vi "averageMeasures.vi"(6 "shift_step_us":dbl=25.0 caption="Shift step", 8 "delay_us":dbl caption="Delay", 9 "repetitions":i32, 11 "counts":u32[][](array[numeric])) -> (2 "delays":dbl[](array[numeric]), 3 "counts":dbl[][](array[numeric]))   [LabVIEW 2014]
uses:
  <vilib>/Analysis/baseanly.llb/Vector x A.vi
  <vilib>/Analysis/Matrix/Numeric/Conversions/Array To Matrix - RA2.vi
  <vilib>/Analysis/Matrix/NI_Matrix.lvlib
  <vilib>/Analysis/NI_AALBase.lvlib
panel:
  out "V' x A":dbl[](array[numeric])
  out "subarray":u32[][](array[numeric])
  out "counts 2":u32[][](array[numeric])
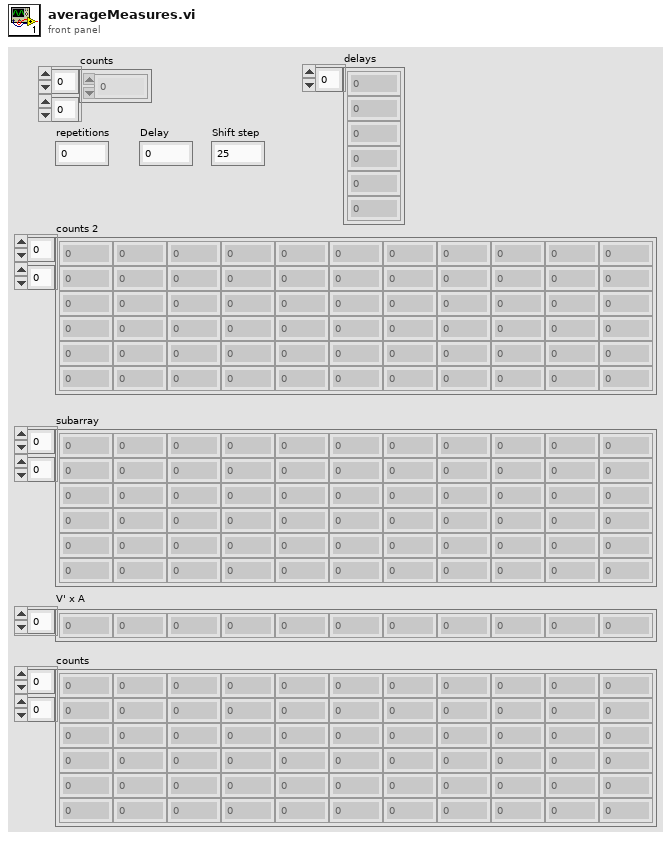
[diagram p1: front panel]
types:
  T1 = typedef "NI_Matrix.lvlib/RealMatrix.ctl" = dbl[][]
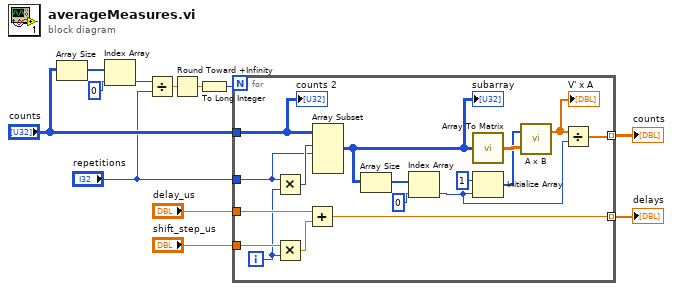
[diagram p0: block diagram]
diagram:
  n1 = Array Size(array="counts") -> (size(s)=w10:i32[])
  n2 = Index Array(array=w10, index=0) -> (element=w6:i32)
  n3 = Divide(x=w6, y="repetitions") -> (x/y=w5:dbl)
  n4 = Round Toward +Infinity(x=w5) -> (ceil(x): smallest int >= x=w2:dbl)
  n5 = To Long Integer(number=w2) -> (32bit integer=w1:i32)
  n6 = for {
    N: w1 -> [_]
    tunnel: "counts" -> [w29]
    tunnel: "repetitions" -> [w20]
    tunnel: "shift_step_us" -> [w28]
    tunnel: "delay_us" -> [w26]
    tunnel: [w17] -> w3 mode=indexing
    tunnel: [w18] -> w4 mode=indexing
    i -> [w19]
    n7 = Multiply(x=w20, y=w19) -> (x*y=w25:i32)
    n8 = Multiply(x=w28, y=w19) -> (x*y=w27:dbl)
    n9 = Add(x=w26, y=w27) -> (x+y=w18:dbl)
    n10 = Array Subset(array=w29, index (row)=w25, length (row)=w20) -> (w16:u32[][])  [unwired: 2 in]
    "subarray" <- w16
    n11 = Array Size(array=w16) -> (size(s)=w15:i32[])
    n12 = Index Array(array=w15, index=0) -> (element=w14:i32)
    n13 = call-poly <vilib>:"Array To Matrix.vi"("Real 2D Array"=w16) -> ("Real Matrix"=w24:T1)
    n14 = Initialize Array(u32 1 ("element"), w14) -> (w22:u32[])
    n15 = call-poly <vilib>:"A x B.vi"("Matrix A"=w24, "Vector V'"=w22) -> ("V' x A"=w21:dbl[])  [unwired: 1 out]
    "V' x A" <- w21
    n16 = Divide(x=w21, y=w14) -> (x/y=w17:dbl[])
    "counts 2" <- w29
  }
  "delays" <- w4
  "counts" <- w3
